vi "Translate passed.vi"(8 "Sprachliste":string[][](array[string]), 9 "Array (Eingang)":string[](array[string])) -> (1 "Array (Ausgang)":string[](array[string]))   [LabVIEW 2020, in "Erweiterte Konfig.lvlib" / "CG-Check Konfig.lvlib"]
uses:
  CG-Check Konfig.lvlib
  Sprachverwaltung/Sprachverwaltung.lvlib
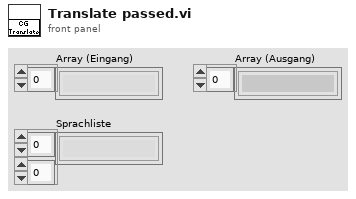
[diagram p1: front panel]
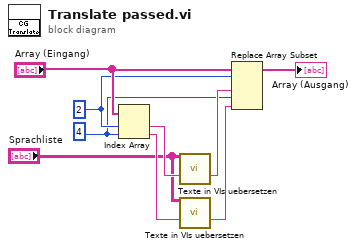
[diagram p0: block diagram]
diagram:
  w2 = 4 ("Index")
  w7 = 2 ("Index")
  n1 = Index Array(array="Array (Eingang)", index #1=w7, index #2=w2) -> (element #1=w5:string, element #2=w4:string)
  n2 = call "Texte in VIs uebersetzen.vi"("Sprachliste"="Sprachliste", "String zum Übersetzen"=w5) -> ("String zum Übersetzen"=w6:string)  [unwired: 9 in, 4 out]
  n3 = call "Texte in VIs uebersetzen.vi"("Sprachliste"="Sprachliste", "String zum Übersetzen"=w4) -> ("String zum Übersetzen"=w1:string)  [unwired: 9 in, 4 out]
  n4 = Replace Array Subset(array="Array (Eingang)", new element #1=w6, index #1=w7, new element #2=w1, index #2=w2) -> (→"Array (Ausgang)":string[])
